vi "Run Inflation Test.vi"(7 "iteration":i32, 8 "error in (no error)":errorcluster, 9 "controller data":T4 {"rectangle"."Rotation" format="%.2f"; "rectangle"."Left" scale=0.0..1024.0; "rectangle"."Right" scale=0.0..1024.0}, 10 "msg network":T3, 11 "start time in":timestamp) -> (0 "error out":errorcluster, 1 "ia test data":T2, 2 "cam timed out?":bool, 3 "start time out":timestamp, 5 "image":T1)   [LabVIEW 2020]
uses:
  Controller Loop/Message and Data.ctl
  Parameter Class/IA Test Parameters.lvclass
  Controllers/Controller.lvclass
  Hardware/Sensors/Cameras/Camera.lvclass
  Hardware/Sensors/Force Sensors/Force Sensor.lvclass
  Hardware/Actuators/Servos/Servo.lvclass
  Hardware/Actuators/Switches/Switch.lvclass
  File Interfacing/Filename Structure.ctl
  Messaging/Messaging Cluster.ctl
  GUI/Main GUI Loop/Handler.ctl
  Result Handling/Inflation Test Numeric Results.ctl
  <vilib>/vision/Image Controls.llb/IMAQ Image.ctl
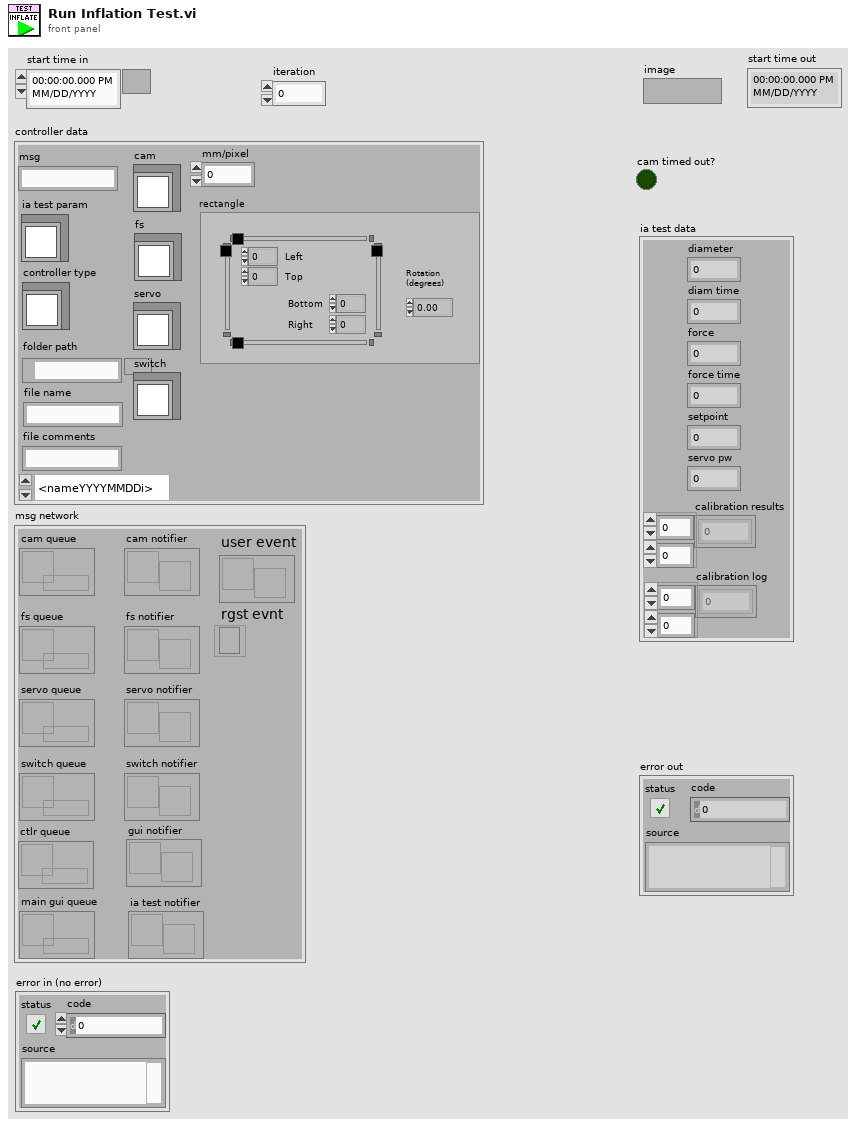
[diagram p1: front panel]
types:
  T1 = typedef "IMAQ Image.ctl" = refnum<image>
  T2 = typedef "Inflation Test Numeric Results.ctl" = cluster{"diameter":dbl, "diam time":dbl, "force":dbl, "force time":dbl, "setpoint":dbl, "servo pw":dbl, "calibration log":dbl[][], "calibration results":dbl[][]}
  T3 = typedef "Messaging Cluster.ctl" = cluster{"cam queue":refnum<queue>, "fs queue":refnum<queue>, "servo queue":refnum<queue>, "switch queue":refnum<queue>, "switch notifier":refnum<notifier>, "servo notifier":refnum<notifier>, "fs notifier":refnum<notifier>, "cam notifier":refnum<notifier>, "rgst evnt":refnum<event-registration>, "user event":refnum<user-event>, "ctlr queue":refnum<queue>, "main gui queue":refnum<queue>, "gui notifier":refnum<notifier>, "ia test notifier":refnum<notifier>}
  T4 = typedef "Message and Data.ctl" = cluster{"msg":string, "ia test param":refnum<class "IA Test Parameters.lvclass">, "controller type":refnum<class "Controller.lvclass">, "folder path":path, "file name":string, "file comments":string, "cam":refnum<class "Camera.lvclass">, "fs":refnum<class "Force Sensor.lvclass">, "servo":refnum<class "Servo.lvclass">, "switch":refnum<class "Switch.lvclass">, "filename struct":T5, "mm/pixel":dbl, "rectangle":T6}
  T5 = typedef "Filename Structure.ctl" = enum16{"<nameYYYYMMDDi>", "<name>"}
  T6 = typedef "IMAQ Rectangle" = cluster{"Left":i32, "Top":i32, "Right":i32, "Bottom":i32, "Rotation":dbl}
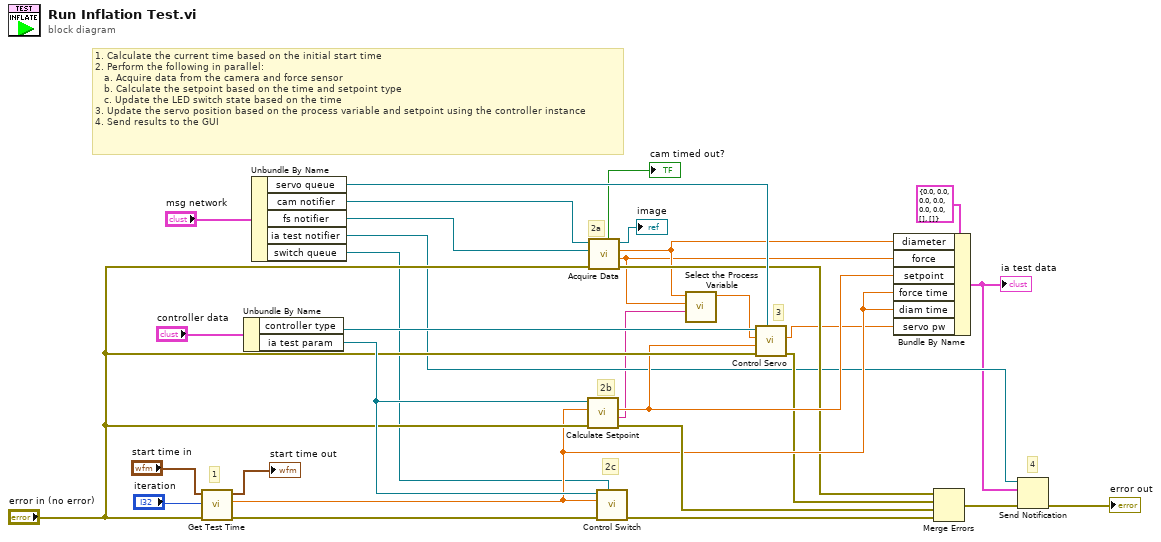
[diagram p0: block diagram]
diagram:
  # "4"
  # "1. Calculate the current time based on the initial start time\n2. Perform the following in parallel:\n   a. Acquire data from the camera and force sensor\n   b. Calculate the setpoint based on the time and setpoint type\n   c. Update the LED switch state based on the time\n3. Update the servo position based on the process variable and setpoint using the controller instance\n4. Send results to the GUI"
  # "2c"
  # "3"
  # "2b"
  # "2a"
  # "1"
  n1 = call "Get Test Time.vi"("error in (no error)"="error in (no error)", "loop iteration"="iteration", "start time in"="start time in") -> ("error out"=w20:errorcluster, "current time"=w15:dbl, "start time out"=→"start time out":timestamp)  [unwired: 6 in]
  n2 = Unbundle By Name("controller data") -> ("controller type"=w31:refnum<class "Controller.lvclass">, "ia test param"=w21:refnum<class "IA Test Parameters.lvclass">)
  n3 = Unbundle By Name("msg network") -> ("servo queue"=w30:refnum<queue>, "cam notifier"=w24:refnum<notifier>, "fs notifier"=w29:refnum<notifier>, "ia test notifier"=w8:refnum<notifier>, "switch queue"=w9:refnum<queue>)
  n4 = call-dynamic "Calculate Setpoint.vi"("error in (no error)"="error in (no error)", "time (sec)"=w15, "IA Test Parameters in"=w21) -> ("error out"=w17:errorcluster, "type"=w4:string, "setpoint"=w16:dbl)  [unwired: 4 in, 2 out]
  n5 = call "Acquire Data.vi"("error in (no error)"="error in (no error)", "fs notifier"=w29, "cam notifier"=w24) -> ("error out"=w11:errorcluster, "force (V)"=w1:dbl, "diameter (mm)"=w3:dbl, "image"=→"image":T1, "cam timed out?"=→"cam timed out?":bool)  [unwired: 4 in]
  n6 = call "Control Switch.vi"("switch queue"=w9, "error in (no error)"=w20, "current time"=w15, "test params"=w21) -> ("error out"=w19:errorcluster)  [unwired: 7 in]
  n7 = call "Select the Process Variable.vi"("type"=w4, "force"=w1, "diameter"=w3) -> ("process variable"=w2:dbl)  [unwired: 8 in]
  n8 = call "Control Servo.vi"("servo queue"=w30, "error in (no error)"="error in (no error)", "setpoint"=w16, "process variable"=w2, "Controller in"=w31) -> ("error out"=w12:errorcluster, "servo pw (us)"=w10:dbl)  [unwired: 5 in]
  n9 = Bundle By Name(cluster=T2 {"diameter"=0.0, "diam time"=0.0, "force"=0.0, "force time"=0.0, "setpoint"=0.0, "servo pw"=0.0, "calibration log"=[], "calibration results"=[]} ("inflation test numeric results"), "diameter"=w3, "force"=w1, "setpoint"=w16, "force time"=w15, "diam time"=w15, "servo pw"=w10) -> (w5:T2)
  "ia test data" <- w5
  n10 = Merge Errors(w11, w12, w17, w19) -> (w7:errorcluster)
  n11 = Send Notification(notification=w5, notifier=w8, error in (no error)=w7) -> (error out=→"error out":errorcluster)  [unwired: 1 out]
